vi "Init Device.vi"(7 "Layout Ref":refnum<vi>, 8 "error in (no error)":errorcluster, 10 "Chan# Array":i32[](array[numeric]), 11 "Device in":refnum<class "Device.lvclass">) -> (0 "error out":errorcluster, 3 "Device out":refnum<class "Device.lvclass">)   [LabVIEW 2013, in "Device.lvclass"]
doc: "Initialize the correct columns and their default appearance.\nUse the front panel to change default appearance of the device in the Add/Manage devices.\n\nOpen a specific device implementation for details."
uses:
  Device.lvclass
panel:
  # "Open a specific devices override of this VI for implementation."
  # "Intended functionality:\n------------------------\nPlace controls here for Device programmer OR advanced user to configure\ntypical layout in the table.\n\nDisplay Info.vi (called on add/manage device) will be where typical user can fine tune."
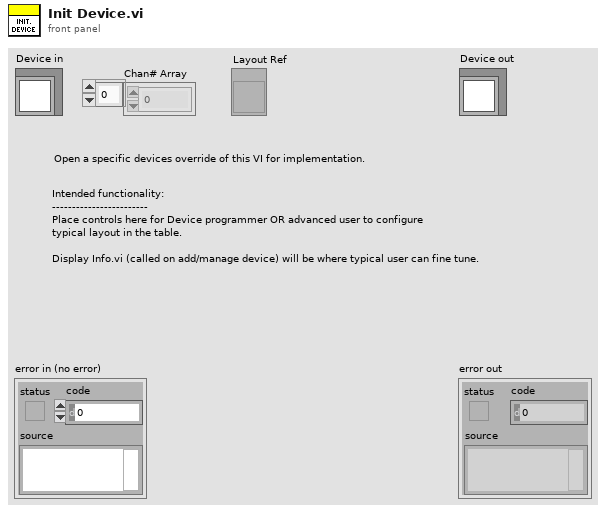
[diagram p1: front panel]
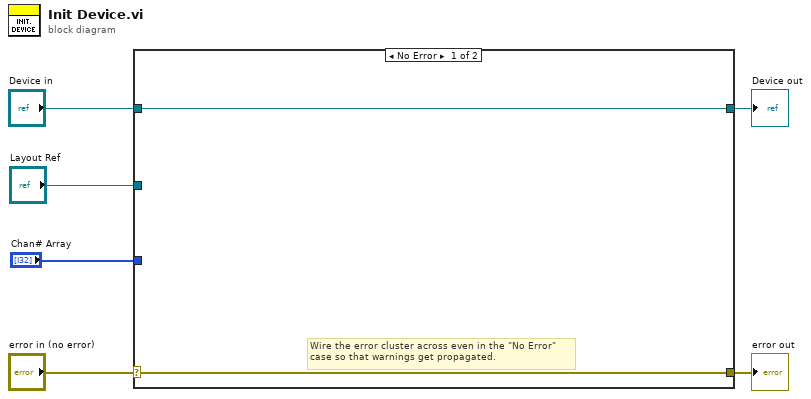
[diagram p0: block diagram]
diagram:
  n1 = case shown="No Error" "error in (no error)" {
    selector: "error in (no error)" -> [w7 w10]
    tunnel: [w7 w10] -> w5
    tunnel: [w8 w9] -> w3
    tunnel: "Device in" -> [w8 w9]
    tunnel: "Layout Ref" -> [_ _]
    tunnel: "Chan# Array" -> [_ _]
    frame No Error {
      # "Wire the error cluster across even in the \"No Error\"\ncase so that warnings get propagated."
    }
    frame Error {
    }
  }
  "error out" <- w5
  "Device out" <- w3
